vi "线性转换.vi"(7 "线性关系":cluster{"X0":dbl, "X1":dbl, "Y0":dbl, "Y1":dbl}, 11 "input":dbl) -> (3 "output":dbl)   [LabVIEW 2016, in "PLC.lvlib"]
uses:
  PLC.lvlib
  <vilib>/Analysis/6fits.llb/Curve Fitting Criteria.ctl
  <vilib>/Analysis/NI_AALPro.lvlib
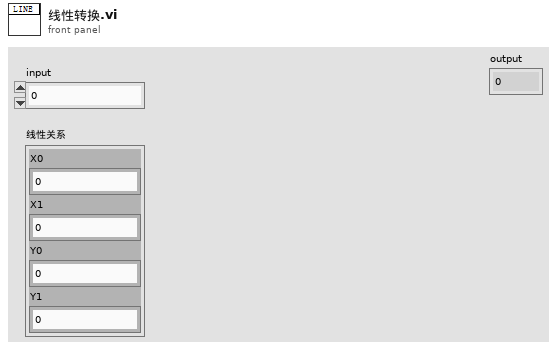
[diagram p1: front panel]
types:
  T1 = typedef "NI_AALPro.lvlib/Curve Fitting Criteria.ctl" = u16
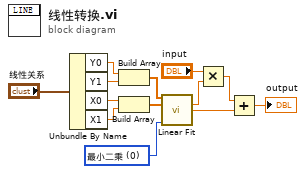
[diagram p0: block diagram]
diagram:
  w13 = T1 0 items=["最小二乘", "最小绝对残差", "Bisquare"] ("method")
  n1 = Unbundle By Name("线性关系") -> ("Y0"=w5:dbl, "Y1"=w6:dbl, "X0"=w3:dbl, "X1"=w2:dbl)
  n2 = Build Array(w5, w6) -> (w4:dbl[])
  n3 = Build Array(w3, w2) -> (w1:dbl[])
  n4 = call <vilib>:"Linear Fit.vi"("Y"=w4, "X"=w1, "method"=w13) -> ("slope"=w11:dbl, "intercept"=w9:dbl)  [unwired: 8 in, 3 out]
  n5 = Multiply(x="input", y=w11) -> (x*y=w10:dbl)
  n6 = Add(x=w10, y=w9) -> (x+y=→"output":dbl)
